vi "dds.vi"() -> ()   [LabVIEW 2020]
uses:
  <vilib>/Platform/TimedLoop/XDataNode/timing_clust.ctl
  <vilib>/Platform/TimedLoop/XDataNode/nitl_modes.ctl
  <vilib>/Platform/TimedLoop/XDataNode/wakeup.ctl
  <instrlib>/_niInstr/DSP/v1/Shared/Public/IQ Data.ctl
  <vilib>/rvi/Emulation/niFpgaGetClockAttributes.vi
  <vilib>/rvi/Emulation/niFpgaSctlEmulationGetInTimedLoop.vi
  <vilib>/rvi/Emulation/niFpgaEmulationReportErrorSimple.vi
  <vilib>/rvi/Emulation/niFpgaCriticalErrorInLSC.vi
  <instrlib>/_niInstr/DSP/v1/FPGA/Public/Sub VIs/Frequency Shift/Frequency Shift - 1 spc.vi
  <vilib>/platform/TimedLoop/XDataNode/XDataNode.xnode
  <instrlib>/_niInstr/DSP/v1/XNodes/Public/Frequency Shift/niInstr DSP v1 Frequency Shift FPGA.xnode
  <vilib>/rvi/FXPMathLib/FxpMul/XNode/nifxpmath_Multiplier.xnode
  <instrlib>/_niInstr/DSP/v1/Shared/niInstr DSP v1 Shared.lvlib
  <instrlib>/_niInstr/DSP/v1/FPGA/niInstr DSP v1 FPGA.lvlib
  <vilib>/Platform/TimedLoop/XDataNode/XDNodeRunTimeDep.lvlib
  <vilib>/rvi/FXPMathLib/sim/FxpSim.dll
panel:
  in  "frequency(kHz) 2":fxp<+,32,16>
  in  "frequency(kHz)":fxp<+,32,16>
  out "single precision float 2":sgl(graph)
  out "single precision float":sgl(graph)
  in  "amplitude":fxp<+/-,16,16>
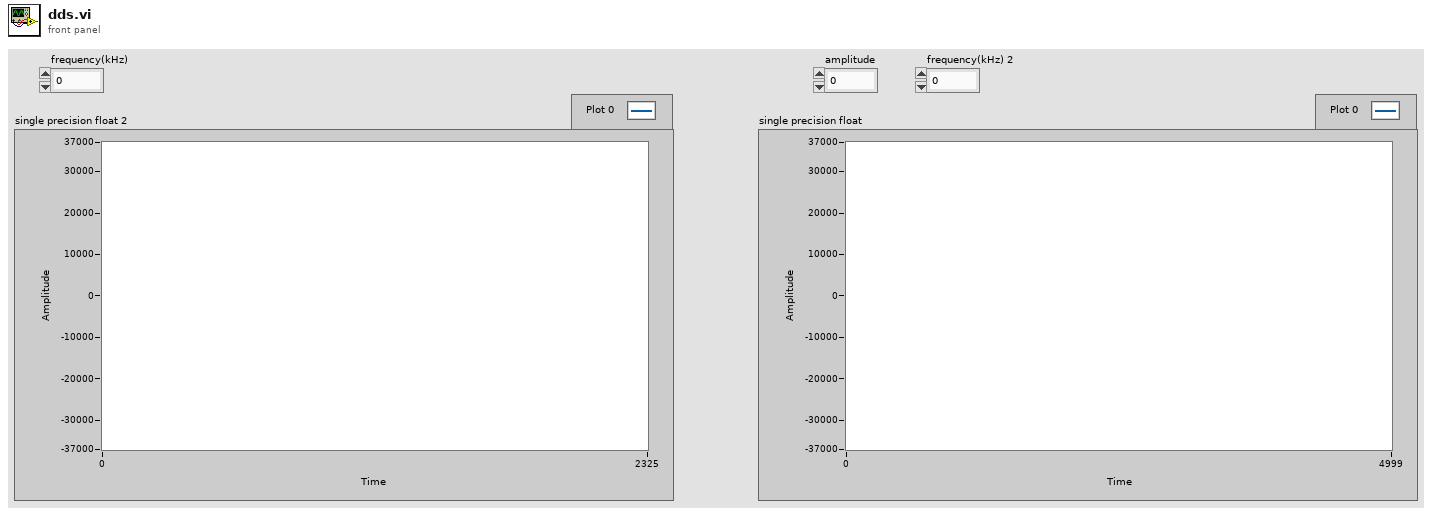
[diagram p1: front panel]
types:
  T1 = typedef "XDNodeRunTimeDep.lvlib/timing_clust.ctl" = cluster{"Expected End [f-1]":u64, "Actual End [f-1]":u64, "Finished Late? [f-1]":bool, "Expected End [i-1]":u64, "Actual End [i-1]":u64, "Finished Late? [i-1]":bool, "Expected Start [i]":u64, "Actual Start [i]":u64, "Expected Start [f]":u64, "Actual Start [f]":u64, "Source Name":string, "Structure Name":string, "Period":i64, "Deadline":i64, "Offset":i64, "Start":i64, "Priority":i32, "Timeout":i32, "Mode":T2, "Wakeup Reason":T3, "Error":errorcluster, "Source Type":string, "Secondary Source Type":string, "Global End Time":u64, "Global Start Time":u64, "Frame Duration":u64, "Iteration Duration":u64, "Assigned CPU":i32, "I/O Scan Engine Mode":u32}
  T2 = typedef "XDNodeRunTimeDep.lvlib/nitl_modes.ctl" = enum32{"No Change", "Process missed periods, maintain original phase", "Discard missed periods, maintain original phase", "Process missed periods, ignore original phase", "Discard missed periods, ignore original phase"}
  T3 = typedef "XDNodeRunTimeDep.lvlib/wakeup.ctl" = enum32{"Normal", "Aborted", "Asynchronous wakeup", "Timing source error", "Timed loop error", "Timeout"}
  T4 = typedef "niInstr DSP v1 Shared.lvlib/IQ Data.ctl" = cluster{"I":fxp<+/-,18,1>, "Q":fxp<+/-,18,1>, "overflow":bool}
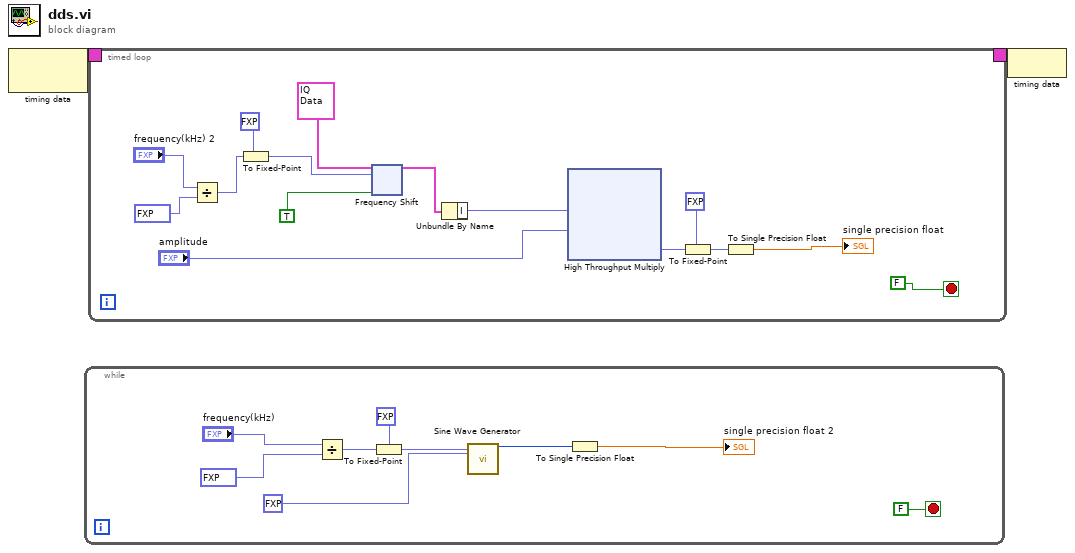
[diagram p0: block diagram]
diagram:
  n1 = node-c288() -> (w2:T1)  [unwired: 1 in]
  n2 = while {
    stop <- FALSE stop-if-true
    n3 = Divide(x="frequency(kHz)", y=fxp<+,32,16> 40000.0 ("frequency (periods/tick)")) -> (x/y=w11:fxp<+,64,32>)
    n4 = To Fixed-Point(fixed-point type=fxp<+,32,0> 0.0 ("frequency (periods/tick)"), number=w11) -> (fixed-point=w8:fxp<+,32,0>)
    n5 = call "Sine Wave Generator"("frequency (periods/tick)"=w8, "phase offset (periods)"=fxp<+,32,0> 0.0) -> ("sine out"=w9:i16)  [unwired: 13 in]
    n6 = To Single Precision Float(number=w9) -> (single precision float=→"single precision float 2":sgl)
  }
  n7 = timed-loop {
    timing: w2 -> [_]
    timing-out: [_] -> w1
    stop <- FALSE stop-if-true
    n8 = Divide(x="frequency(kHz) 2", y=fxp<+,32,16> 40000.0 ("frequency (periods/tick)")) -> (x/y=w14:fxp<+,64,32>)
    n9 = To Fixed-Point(fixed-point type=fxp<+/-,48,0> 0.0 ("frequency shift"), number=w14) -> (fixed-point=w15:fxp<+/-,48,0>)
    n10 = xnode "Frequency Shift"("data in"=T4 {"I"=0.9999923706054688, "Q"=0.0, "overflow"=FALSE}, "frequency shift"=w15, "input valid"=TRUE) -> ("data out"=w26:T4)  [unwired: 3 in, 2 out]
    n11 = Unbundle By Name(w26) -> ("I"=w25:fxp<+/-,18,1>)
    n12 = xnode "High Throughput Multiply"("x"=w25, "y"="amplitude") -> ("x*y"=w22:fxp<+/-,34,17>)
    n13 = To Fixed-Point(fixed-point type=fxp<+/-,16,16> 0.0, number=w22) -> (fixed-point=w13:fxp<+/-,16,16>)
    n14 = To Single Precision Float(number=w13) -> (single precision float=→"single precision float":sgl)
  }
  n15 = node-c288(w1) -> ()
